vi "Traffic Light.vi"() -> ()   [LabVIEW 2013]
doc: "This Vi is a simulation of Traffic light controller which provides \n-Green\n-Yellow\n-Red light for each direction.\n\nthe period of time for which the light will be On is\n-Green: 4sec\n-Yellow: 2sec\n-Red: 4 sec\nPattern of light will be-\nNorth South East West\nG G R R R-RED, G-GREEN, Y-YELLOW\nY Y R R E-East, W-West, N-North, S-South.\nR R G G\nR R Y Y\n\n\nIf the vehicle present sensor is pressed then the pattern of light will be-\nFor EW sensor-\nNorth South East West\nG G R R R-RED, G-GREEN, Y-YELLOW\nY Y R R E-East, W-West, N-North, S-South.\nR R LG LG\nR R LY LY\nFor NS sensor-\nR R G G\nR R Y Y\nLG LG R R\nLY LY R R"
uses:
  Controls/Traffic light.ctl
  Controls/Traffic_light_left.ctl
  Controls/Traffi Light States.ctl
  Controls/Traffic Signal States.ctl
panel:
  in  "North  Sensor":bool
  in  "Start":bool caption="stop"
  out "South Bound Left":T1
  out "South Bound":T2={"R"=TRUE, "Y"=FALSE, "G"=FALSE}
  out "West Bound Left":T1
  out "West Bound":T2={"R"=TRUE, "Y"=FALSE, "G"=FALSE}
  out "East Bound Left":T1
  out "East Bound":T2={"R"=TRUE, "Y"=FALSE, "G"=FALSE}
  in  "stop":bool
  in  "West Sensor":bool
  in  "East Sensor":bool
  in  "South Sensor":bool
  out "North Bound Left":T1
  out "North Bound":T2={"R"=TRUE, "Y"=FALSE, "G"=FALSE}
  # "-Pattern of light will be(Without sensor)-\nNorth           South              East                West\nG                      G                    R                      R                             R-RED, G-GREEN, Y-YELLOW\nY                       Y                    R                      R                            E-East, W-West, N-North, S-South.\nR                       R                    G                     G\nR                       R                    Y                      Y\n-If the vehicle present sensor is pressed then the pattern of light will be-\n-For EW sensor-\nNorth           South              East                West\nG                      G                    R                      R                             \nY                       Y                    R                      R                            \nR                       R                    LG                     LG\nR                       R                    LY                      LY\n-For NS sensor-\nR                       R                      G                       G\nR                       R                      Y                        Y\nLG                    LG                     R                       R\nLY                    LY                     R                        R"
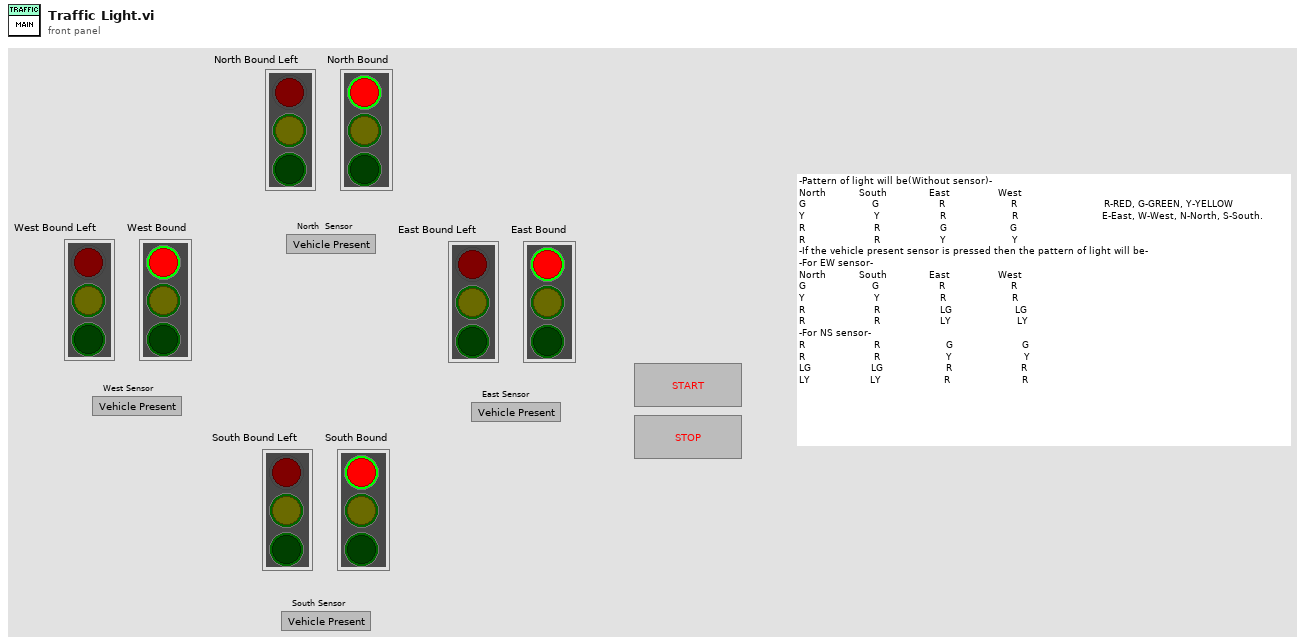
[diagram p1: front panel]
types:
  T1 = typedef "Traffic_light_left.ctl" = cluster{"R":bool, "Y":bool, "G":bool}
  T2 = typedef "Traffic light.ctl" = cluster{"R":bool, "Y":bool, "G":bool}
  T3 = typedef "Traffic Signal States.ctl" = enum16{"NS Green", "NS Yellow", "EW Green", "EW Yellow", "NS Left Green", "NS Left Yellow", "EW Left Green", "EW Left Yellow"}
  T4 = cluster{"North Bound Left":T1, "South Bound Left":T1, "East Bound Left":T1, "West Bound Left":T1, "North Bound":T2, "South Bound":T2, "East Bound":T2, "West Bound":T2}
  T5 = typedef "Traffi Light States.ctl" = enum16{"Initialize", "Main", "Stop"}
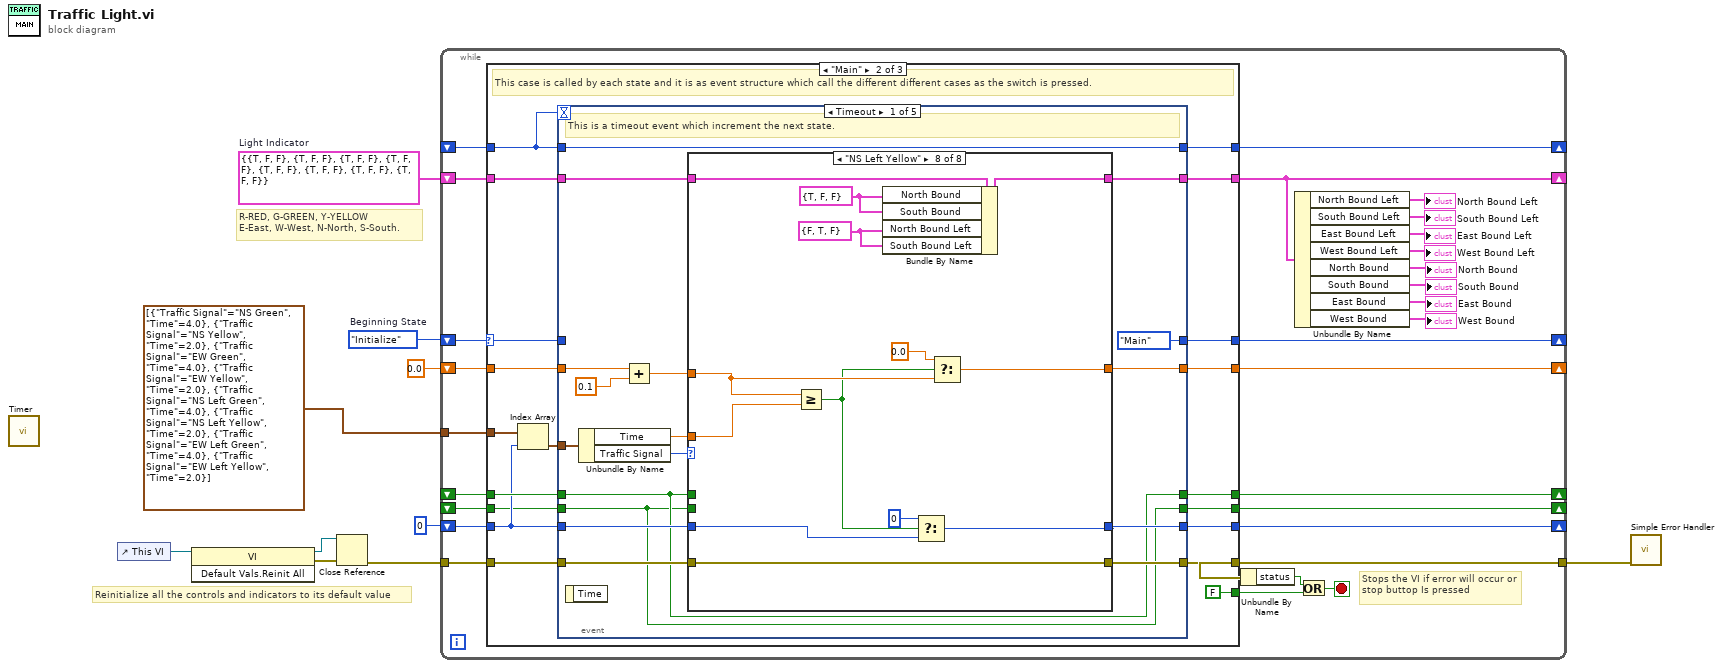
[diagram p0: block diagram]
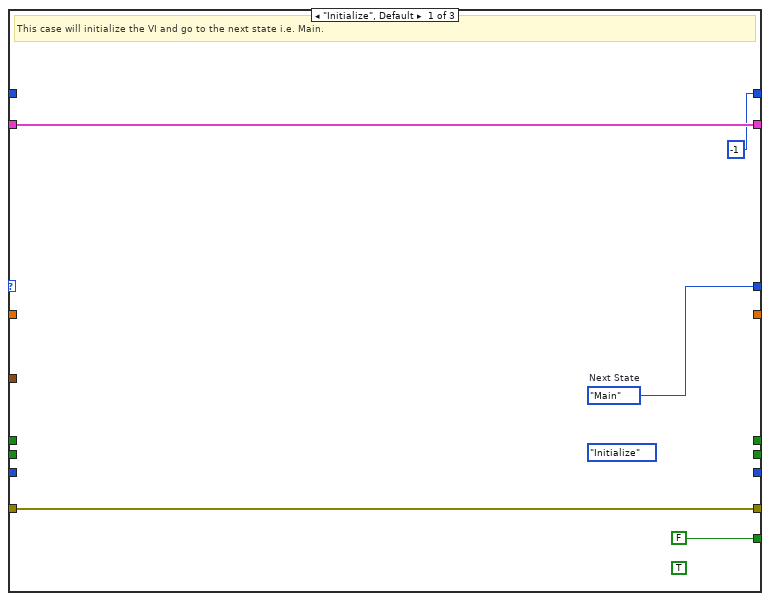
[diagram p2: hidden frame]
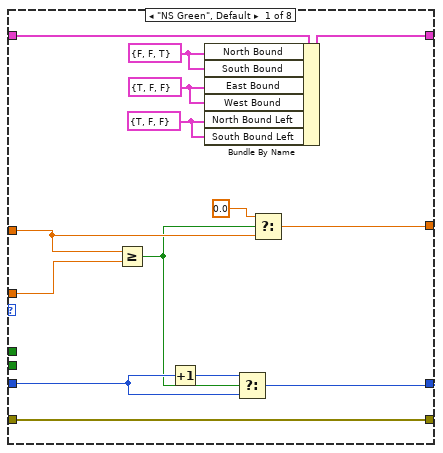
[diagram p3: hidden frame]
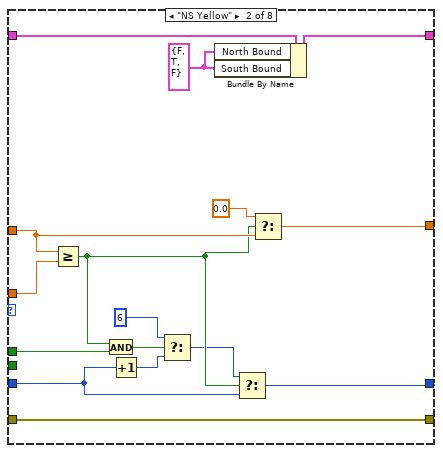
[diagram p4: hidden frame]
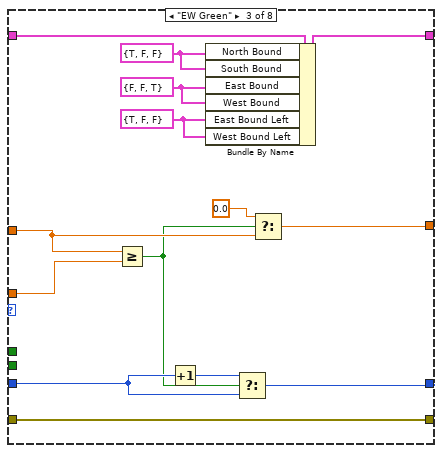
[diagram p5: hidden frame]
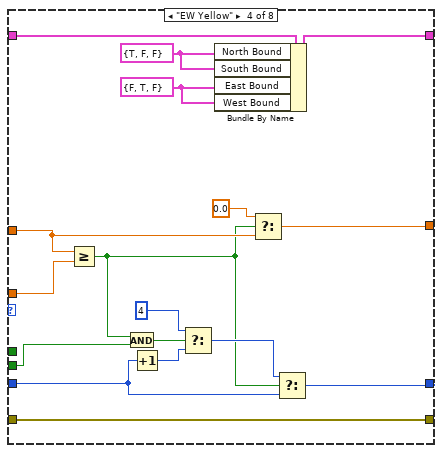
[diagram p6: hidden frame]
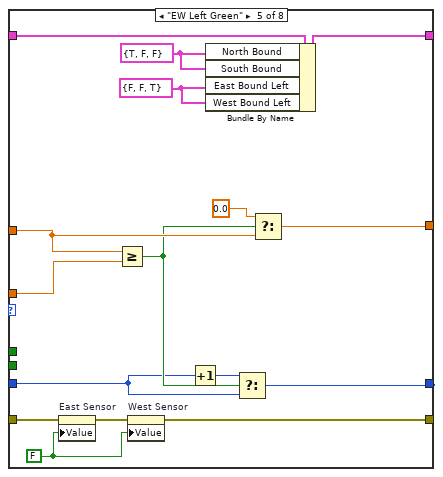
[diagram p7: hidden frame]
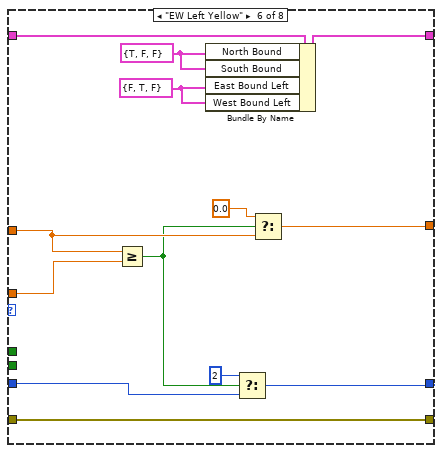
[diagram p8: hidden frame]
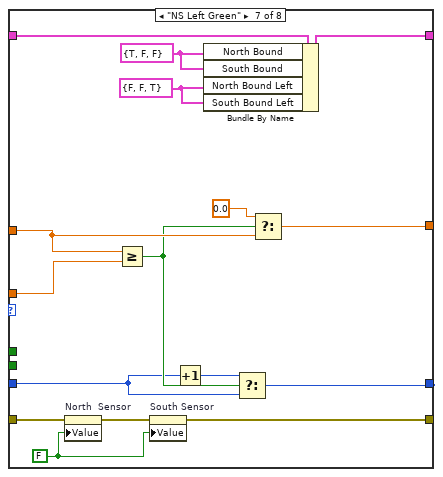
[diagram p9: hidden frame]
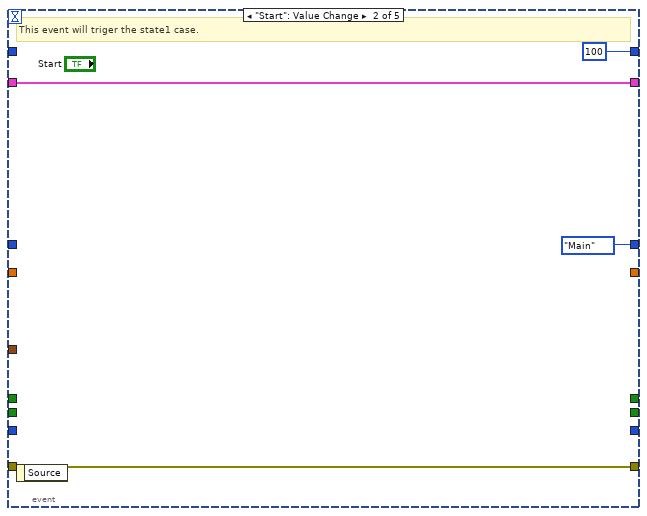
[diagram p10: hidden frame]
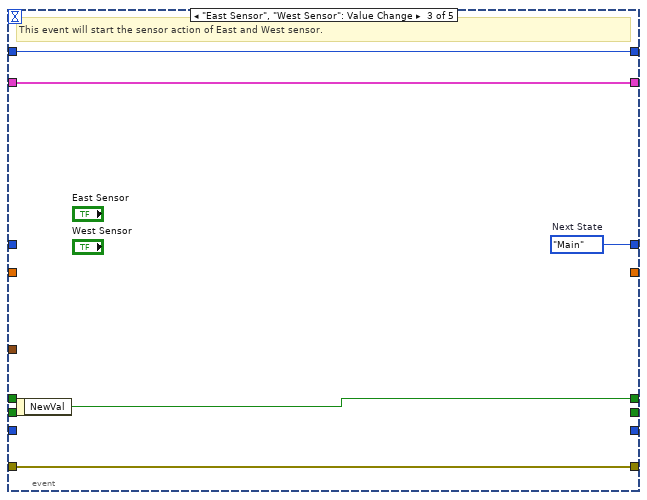
[diagram p11: hidden frame]
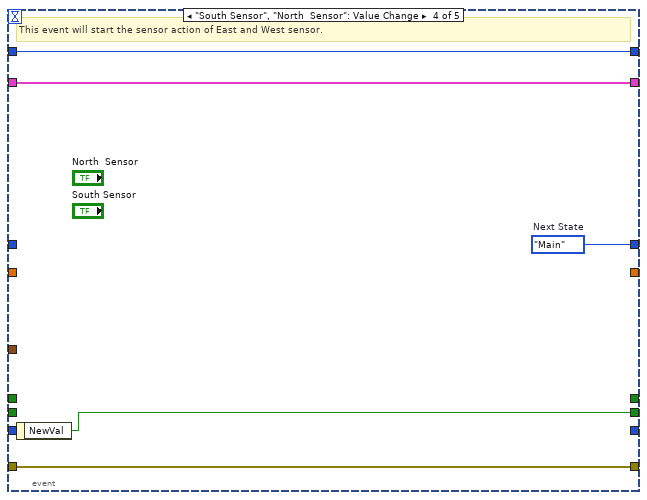
[diagram p12: hidden frame]
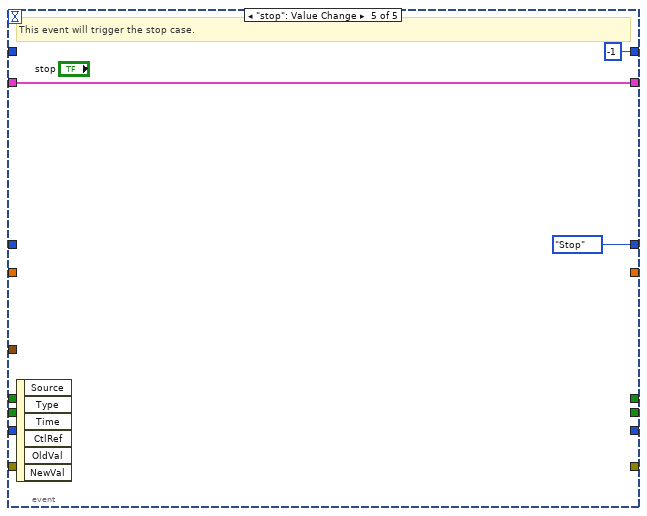
[diagram p13: hidden frame]
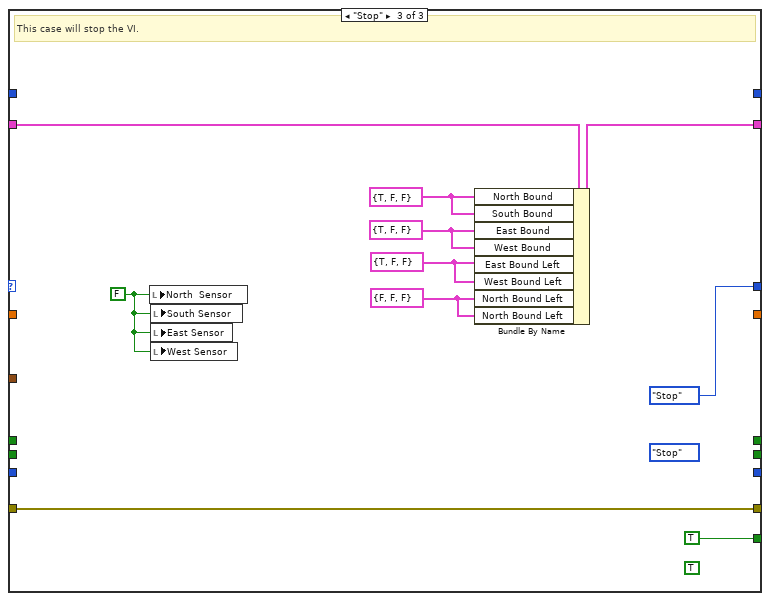
[diagram p14: hidden frame]
diagram:
  w4 = T4 {"North Bound Left"={"R"=TRUE, "Y"=FALSE, "G"=FALSE}, "South Bound Left"={"R"=TRUE, "Y"=FALSE, "G"=FALSE}, "East Bound Left"={"R"=TRUE, "Y"=FALSE, "G"=FALSE}, "West Bound Left"={"R"=TRUE, "Y"=FALSE, "G"=FALSE}, "North Bound"={"R"=TRUE, "Y"=FALSE, "G"=FALSE}, "South Bound"={"R"=TRUE, "Y"=FALSE, "G"=FALSE}, "East Bound"={"R"=TRUE, "Y"=FALSE, "G"=FALSE}, "West Bound"={"R"=TRUE, "Y"=FALSE, "G"=FALSE}}  # Light Indicator
  w10 = Traffi_Light_States."Initialize"  # Beginning State
  # "R-RED, G-GREEN, Y-YELLOW\nE-East, W-West, N-North, S-South."
  # "Reinitialize all the controls and indicators to its default value"
  n1 = call "Timer.vi"() -> ()  [unwired: 9 in, 3 out]
  n2 = control-ref of="This VI"() -> (w9:refnum<vi>)
  n3 = invoke class="VI" method="Default Vals.Reinit All"(reference=w9) -> (reference out=w7:refnum<vi>, error out=w8:errorcluster)  [unwired: 2 in, 1 out]
  n4 = Close Reference(reference=w7, error in (no error)=w8) -> (error out=w6:errorcluster)
  n5 = while {
    shift-right: [w37] -> _
    shift-left: w10 -> [w38]
    tunnel: w6 -> [w36]
    tunnel: [w35] -> w5
    shift-right: [w22] -> _
    shift-left: w4 -> [w31]
    shift-right: [w21] -> _
    shift-left: _ -> [w20]
    tunnel: cluster{"Traffic Signal":T3, "Time":dbl}[] [{"Traffic Signal"=enum."NS Green", "Time"=4.0}, {"Traffic Signal"=enum."NS Yellow", "Time"=2.0}, {"Traffic Signal"=enum."EW Green", "Time"=4.0}, {"Traffic Signal"=enum."EW Yellow", "Time"=2.0}, {"Traffic Signal"=enum."NS Left Green", "Time"=4.0}, {"Traffic Signal"=enum."NS Left Yellow", "Time"=2.0}, {"Traffic Signal"=enum."EW Left Green", "Time"=4.0}, {"Traffic Signal"=enum."EW Left Yellow", "Time"=2.0}] -> [w19]
    shift-right: [w17] -> _
    shift-left: 0.0 -> [w18]
    shift-right: [w16] -> _
    shift-left: 0 -> [w15]
    shift-right: [w14] -> _
    shift-left: _ -> [w13]
    shift-right: [w12] -> _
    shift-left: _ -> [w11]
    stop <- w34 stop-if-true
    # "Stops the VI if error will occur or stop buttop Is pressed"
    n6 = case shown="\"Main\"" w38 {
      selector: w38 -> [_ w56 _]
      tunnel: [w43 w57 Traffi_Light_States."Stop" ("f")] -> w37
      tunnel: w36 -> [w42 w59 w223]
      tunnel: [w42 w58 w223] -> w35
      tunnel: [FALSE FALSE TRUE] -> w32
      tunnel: [w40 w60 w224] -> w22
      tunnel: w31 -> [w40 w61 w225]
      tunnel: [-1 w55 _] -> w21
      tunnel: w20 -> [_ w50 _]
      tunnel: w19 -> [_ w54 _]
      tunnel: w18 -> [_ w52 _]
      tunnel: [_ w51 _] -> w17
      tunnel: [_ w49 _] -> w16
      tunnel: w15 -> [_ w46 _]
      tunnel: [_ w48 _] -> w14
      tunnel: w13 -> [_ w47 _]
      tunnel: [_ w45 _] -> w12
      tunnel: w11 -> [_ w44 _]
      frame "Initialize", Default {
        (unwired) Traffi_Light_States."Initialize" ("f")
        (unwired) TRUE
        w43 = Traffi_Light_States."Main"  # Next State
        # "This case will initialize the VI and go to the next state i.e. Main."
      }
      frame "Main" {
        # "This case is called by each state and it is as event structure which call the different different cases as the switch is pressed."
        n7 = Index Array(array=w54, index=w46) -> (element=w53:cluster{"Traffic Signal":T3, "Time":dbl})
        n8 = event shown="[0] Timeout" {
          selector: _ -> [_ _ _ _ _]
          dyn-events: _ -> [_ _ _ _ _]
          timeout: w50 -> [_ _ _ _ _]
          tunnel: w61 -> [w77 w201 w207 w212 w213]
          tunnel: [w76 w201 w207 w212 w213] -> w60
          tunnel: w59 -> [w72 w200 w206 w211 _]
          tunnel: [w73 w200 w206 w211 _] -> w58
          tunnel: [Traffi_Light_States."Main" Traffi_Light_States."Main" ("Next State") w205 w210 Traffi_Light_States."Stop"] -> w57
          tunnel: w56 -> [_ _ _ _ _]
          tunnel: [w79 100 w204 w209 -1] -> w55
          tunnel: w50 -> [w79 _ w204 w209 _]
          tunnel: w53 -> [w75 _ _ _ _]
          tunnel: w52 -> [w71 _ _ _ _]
          tunnel: [w68 _ _ _ _] -> w51
          tunnel: [w67 _ _ _ _] -> w49
          tunnel: w46 -> [w66 _ _ _ _]
          tunnel: [w64 _ w203 _ _] -> w48
          tunnel: w47 -> [w64 _ _ _ _]
          tunnel: [w63 _ _ w208 _] -> w45
          tunnel: w44 -> [w63 _ _ _ _]
          event Timeout {
            # "This is a timeout event which increment the next state."
            n9 = event-data() -> ()  [unwired: 1 in, 1 out]
            n10 = Unbundle By Name(w75) -> ("Time"=w65:dbl, "Traffic Signal"=w74:T3)
            n11 = Add(x=w71, y=0.1) -> (x+y=w70:dbl)
            n12 = case shown="\"NS Left Yellow\"" w74 {
              tunnel: w77 -> [w93 w109 w123 w140 w156 w169 w185 w198]
              tunnel: [w91 w107 w121 w138 w155 w167 w184 w196] -> w76
              tunnel: [w92 w108 w122 w139 w142 w168 w171 w197] -> w73
              tunnel: w72 -> [w92 w108 w122 w139 w144 w168 w173 w197]
              tunnel: w70 -> [w89 w105 w119 w136 w153 w165 w182 w194]
              tunnel: [w84 w102 w114 w133 w150 w162 w179 w191] -> w68
              tunnel: [w87 w103 w117 w134 w151 w163 w180 w192] -> w67
              tunnel: w66 -> [w86 w96 w116 w125 w146 w158 w175 w187]
              tunnel: w65 -> [w88 w104 w118 w135 w152 w164 w181 w193]
              tunnel: w64 -> [_ w98 _ _ _ _ _ _]
              tunnel: w63 -> [_ _ _ w127 _ _ _ _]
              frame "NS Green", Default {
                w80 = T1 {"R"=TRUE, "Y"=FALSE, "G"=FALSE} ("East Bound Left")
                w81 = T2 {"R"=TRUE, "Y"=FALSE, "G"=FALSE} ("East Bound")
                w90 = T2 {"R"=FALSE, "Y"=FALSE, "G"=TRUE} ("North Bound")
                n13 = Greater Or Equal?(x=w89, y=w88) -> (x >= y?=w83:bool)
                n14 = Increment(x=w86) -> (x+1=w85:i32)
                n15 = Bundle By Name(cluster=w93, "North Bound"=w90, "South Bound"=w90, "East Bound"=w81, "West Bound"=w81, "North Bound Left"=w80, "South Bound Left"=w80) -> (w91:T4)
                n16 = Select(t=w85, s=w83, f=w86) -> (s? t:f=w87:i32)
                n17 = Select(t=0.0, s=w83, f=w89) -> (s? t:f=w84:dbl)
              }
              frame "NS Yellow" {
                w106 = T2 {"R"=FALSE, "Y"=TRUE, "G"=FALSE} ("North Bound")
                n18 = Greater Or Equal?(x=w105, y=w104) -> (x >= y?=w99:bool)
                n19 = And(x=w99, y=w98) -> (x .and. y?=w97:bool)
                n20 = Increment(x=w96) -> (x+1=w95:i32)
                n21 = Select(t=6, s=w97, f=w95) -> (s? t:f=w94:i32)
                n22 = Bundle By Name(cluster=w109, "North Bound"=w106, "South Bound"=w106) -> (w107:T4)
                n23 = Select(t=w94, s=w99, f=w96) -> (s? t:f=w103:i32)
                n24 = Select(t=0.0, s=w99, f=w105) -> (s? t:f=w102:dbl)
              }
              frame "EW Green" {
                w110 = T1 {"R"=TRUE, "Y"=FALSE, "G"=FALSE} ("East Bound Left")
                w111 = T2 {"R"=FALSE, "Y"=FALSE, "G"=TRUE} ("East Bound")
                w120 = T2 {"R"=TRUE, "Y"=FALSE, "G"=FALSE} ("North Bound")
                n25 = Greater Or Equal?(x=w119, y=w118) -> (x >= y?=w113:bool)
                n26 = Increment(x=w116) -> (x+1=w115:i32)
                n27 = Bundle By Name(cluster=w123, "North Bound"=w120, "South Bound"=w120, "East Bound"=w111, "West Bound"=w111, "East Bound Left"=w110, "West Bound Left"=w110) -> (w121:T4)
                n28 = Select(t=w115, s=w113, f=w116) -> (s? t:f=w117:i32)
                n29 = Select(t=0.0, s=w113, f=w119) -> (s? t:f=w114:dbl)
              }
              frame "EW Yellow" {
                w131 = T2 {"R"=FALSE, "Y"=TRUE, "G"=FALSE} ("East Bound")
                w137 = T2 {"R"=TRUE, "Y"=FALSE, "G"=FALSE} ("North Bound")
                n30 = Greater Or Equal?(x=w136, y=w135) -> (x >= y?=w124:bool)
                n31 = And(x=w124, y=w127) -> (x .and. y?=w129:bool)
                n32 = Increment(x=w125) -> (x+1=w128:i32)
                n33 = Select(t=4, s=w129, f=w128) -> (s? t:f=w126:i32)
                n34 = Bundle By Name(cluster=w140, "North Bound"=w137, "South Bound"=w137, "East Bound"=w131, "West Bound"=w131) -> (w138:T4)
                n35 = Select(t=0.0, s=w124, f=w136) -> (s? t:f=w133:dbl)
                n36 = Select(t=w126, s=w124, f=w125) -> (s? t:f=w134:i32)
              }
              frame "EW Left Green" {
                w141 = FALSE ("East Sensor")
                w147 = T1 {"R"=FALSE, "Y"=FALSE, "G"=TRUE} ("North Bound Left")
                w154 = T2 {"R"=TRUE, "Y"=FALSE, "G"=FALSE} ("North Bound")
                n37 = property on="East Sensor" class="Bool (strict)"(error in=w144, "Value"=w141) -> (error out=w143:errorcluster)  [unwired: 1 in, 1 out]
                n38 = Greater Or Equal?(x=w153, y=w152) -> (x >= y?=w149:bool)
                n39 = property on="West Sensor" class="Bool (strict)"(error in=w143, "Value"=w141) -> (error out=w142:errorcluster)  [unwired: 1 in, 1 out]
                n40 = Increment(x=w146) -> (x+1=w145:i32)
                n41 = Bundle By Name(cluster=w156, "North Bound"=w154, "South Bound"=w154, "East Bound Left"=w147, "West Bound Left"=w147) -> (w155:T4)
                n42 = Select(t=w145, s=w149, f=w146) -> (s? t:f=w151:i32)
                n43 = Select(t=0.0, s=w149, f=w153) -> (s? t:f=w150:dbl)
              }
              frame "EW Left Yellow" {
                w159 = T1 {"R"=FALSE, "Y"=TRUE, "G"=FALSE} ("North Bound Left")
                w166 = T2 {"R"=TRUE, "Y"=FALSE, "G"=FALSE} ("North Bound")
                n44 = Greater Or Equal?(x=w165, y=w164) -> (x >= y?=w161:bool)
                n45 = Bundle By Name(cluster=w169, "North Bound"=w166, "South Bound"=w166, "East Bound Left"=w159, "West Bound Left"=w159) -> (w167:T4)
                n46 = Select(t=2, s=w161, f=w158) -> (s? t:f=w163:i32)
                n47 = Select(t=0.0, s=w161, f=w165) -> (s? t:f=w162:dbl)
              }
              frame "NS Left Green" {
                w170 = FALSE ("North  Sensor")
                w176 = T1 {"R"=FALSE, "Y"=FALSE, "G"=TRUE} ("North Bound Left")
                w183 = T2 {"R"=TRUE, "Y"=FALSE, "G"=FALSE} ("North Bound")
                n48 = property on="North  Sensor" class="Bool (strict)"(error in=w173, "Value"=w170) -> (error out=w172:errorcluster)  [unwired: 1 in, 1 out]
                n49 = Greater Or Equal?(x=w182, y=w181) -> (x >= y?=w178:bool)
                n50 = property on="South Sensor" class="Bool (strict)"(error in=w172, "Value"=w170) -> (error out=w171:errorcluster)  [unwired: 1 in, 1 out]
                n51 = Increment(x=w175) -> (x+1=w174:i32)
                n52 = Bundle By Name(cluster=w185, "North Bound"=w183, "South Bound"=w183, "North Bound Left"=w176, "South Bound Left"=w176) -> (w184:T4)
                n53 = Select(t=w174, s=w178, f=w175) -> (s? t:f=w180:i32)
                n54 = Select(t=0.0, s=w178, f=w182) -> (s? t:f=w179:dbl)
              }
              frame "NS Left Yellow" {
                w188 = T1 {"R"=FALSE, "Y"=TRUE, "G"=FALSE} ("North Bound Left")
                w195 = T2 {"R"=TRUE, "Y"=FALSE, "G"=FALSE} ("North Bound")
                n55 = Greater Or Equal?(x=w194, y=w193) -> (x >= y?=w190:bool)
                n56 = Bundle By Name(cluster=w198, "North Bound"=w195, "South Bound"=w195, "North Bound Left"=w188, "South Bound Left"=w188) -> (w196:T4)
                n57 = Select(t=0, s=w190, f=w187) -> (s? t:f=w192:i32)
                n58 = Select(t=0.0, s=w190, f=w194) -> (s? t:f=w191:dbl)
              }
            }
          }
          event "Start": Value Change {
            # "This event will triger the state1 case."
            n59 = event-data() -> ()  [unwired: 1 in, 1 out]
          }
          event "East Sensor", "West Sensor": Value Change {
            w205 = Traffi_Light_States."Main"  # Next State
            # "This event will start the sensor action of East and West sensor."
            n60 = event-data() -> ("NewVal"=w203:bool)  [unwired: 1 in]
          }
          event "South Sensor", "North  Sensor": Value Change {
            w210 = Traffi_Light_States."Main"  # Next State
            # "This event will start the sensor action of East and West sensor."
            n61 = event-data() -> ("NewVal"=w208:bool)  [unwired: 1 in]
          }
          event "stop": Value Change {
            # "This event will trigger the stop case."
            n62 = event-data() -> ()  [unwired: 1 in, 6 out]
          }
        }
      }
      frame "Stop" {
        (unwired) TRUE ("Elapsed?")
        w218 = FALSE ("North  Sensor")
        (unwired) Traffi_Light_States."Stop" ("f")
        w219 = T1 {"R"=FALSE, "Y"=FALSE, "G"=FALSE} ("North Bound Left")
        w220 = T1 {"R"=TRUE, "Y"=FALSE, "G"=FALSE} ("East Bound Left")
        w221 = T2 {"R"=TRUE, "Y"=FALSE, "G"=FALSE} ("East Bound")
        w222 = T2 {"R"=TRUE, "Y"=FALSE, "G"=FALSE} ("North Bound")
        # "This case will stop the VI."
        n63 = local write "North  Sensor"(w218) -> ()
        n64 = local write "South Sensor"(w218) -> ()
        n65 = local write "East Sensor"(w218) -> ()
        n66 = local write "West Sensor"(w218) -> ()
        n67 = Bundle By Name(cluster=w225, "North Bound"=w222, "South Bound"=w222, "East Bound"=w221, "West Bound"=w221, "East Bound Left"=w220, "West Bound Left"=w220, "North Bound Left"=w219, "North Bound Left"=w219) -> (w224:T4)
      }
    }
    n68 = Unbundle By Name(w35) -> ("status"=w33:bool)
    n69 = Unbundle By Name(w22) -> ("North Bound Left"=→"North Bound Left":T1, "South Bound Left"=→"South Bound Left":T1, "East Bound Left"=→"East Bound Left":T1, "West Bound Left"=→"West Bound Left":T1, "North Bound"=→"North Bound":T2, "South Bound"=→"South Bound":T2, "East Bound"=→"East Bound":T2, "West Bound"=→"West Bound":T2)
    n70 = Or(x=w33, y=w32) -> (x .or. y?=w34:bool)
  }
  n71 = call <vilib>:"Simple Error Handler.vi"("error in (no error)"=w5) -> ()  [unwired: 4 in, 5 out]
